vi "Set IConfiguration.vi"(8 "error in":errorcluster, 10 "IConfiguration":refnum<class "IConfiguration.lvclass">, 11 "SimpleCsvDataLogger in":refnum<class "SimpleCsvDataLogger.lvclass">) -> (0 "error out":errorcluster, 3 "SimpleCsvDataLogger out":refnum<class "SimpleCsvDataLogger.lvclass">)   [LabVIEW 2019, in "SimpleCsvDataLogger.lvclass"]
uses:
  SimpleCsvDataLogger.lvclass
  SimpleCsvDataLogger.lvclass/SimpleCsvDataLogger.ctl
  Interfaces/IConfiguration/IConfiguration.lvclass
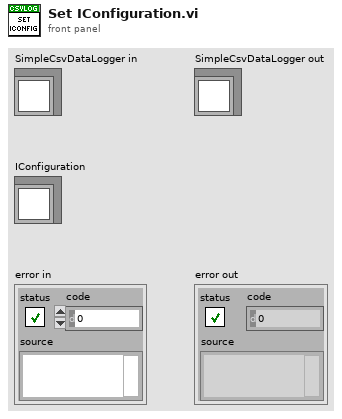
[diagram p1: front panel]
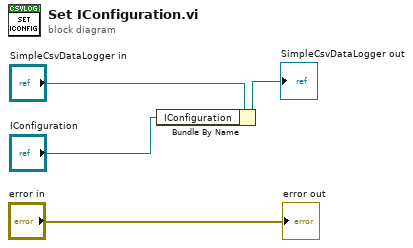
[diagram p0: block diagram]
diagram:
  n1 = Bundle By Name(cluster="SimpleCsvDataLogger in", "IConfiguration"="IConfiguration") -> (→"SimpleCsvDataLogger out":refnum<class "SimpleCsvDataLogger.lvclass">)
  "error out" <- "error in"
